vi "_Get App Ref from Info.vi"(8 "error in (no error)":errorcluster, 9 "Analysis App Info":T1) -> (0 "error out":errorcluster, 1 "Analysis App ref":refnum<vi>)   [LabVIEW 2017, in "CSM_ExampleBrowser.lvlib"]
uses:
  <vilib>/addons/analyzer/_analyzerctrls.llb/VIAnCtl Analysis App Info.ctl
  globals/User Visible Strings.vi
  CSM_ExampleBrowser.lvlib
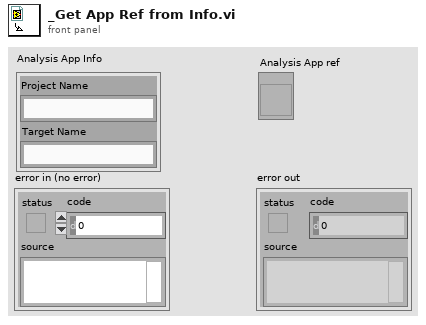
[diagram p1: front panel]
types:
  T1 = typedef "VIAnCtl Analysis App Info.ctl" = cluster{"Project Name":string, "Target Name":string}
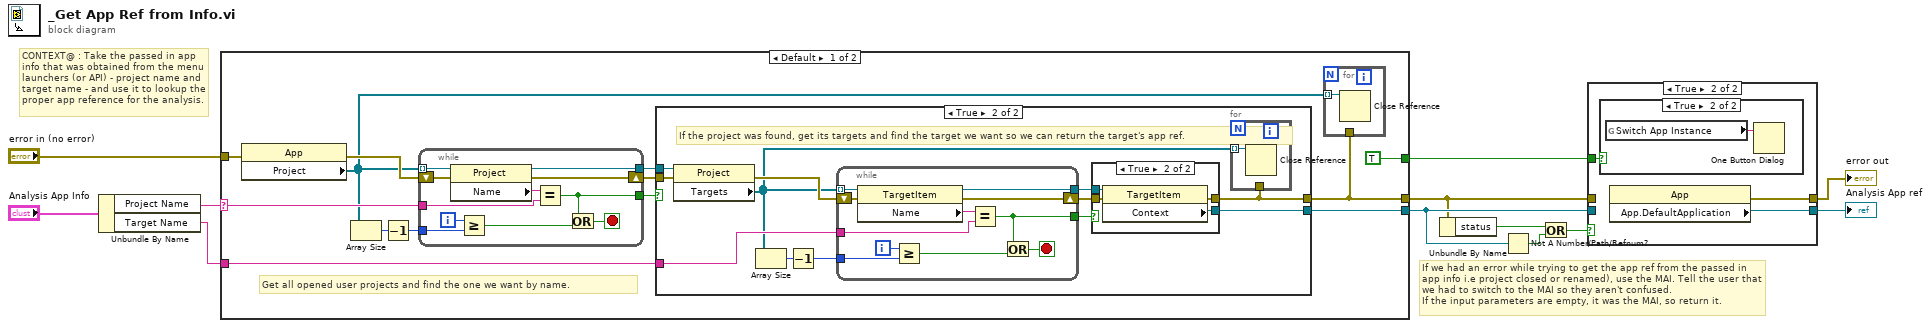
[diagram p0: block diagram]
diagram:
  # "If we had an error while trying to get the app ref from the passed in app info i.e project closed or renamed), use the MAI. Tell the user that we had to switch to the MAI so they aren't confused. \nIf the input parameters are empty, it was the MAI, so return it."
  # "CONTEXT@ : Take the passed in app info that was obtained from the menu launchers (or API) - project name and target name - and use it to lookup the proper app reference for the analysis."
  n1 = Unbundle By Name("Analysis App Info") -> ("Project Name"=w11:string, "Target Name"=w10:string)
  n2 = case shown="Default" w11 {
    selector: w11 -> [w22 _]
    tunnel: [w18 _] -> w6
    tunnel: w10 -> [w19 _]
    tunnel: [w14 _] -> w4
    tunnel: "error in (no error)" -> [w16 _]
    tunnel: [TRUE _] -> w1
    frame Default {
      # "Get all opened user projects and find the one we want by name."
      n3 = property class="App"(error in=w16) -> (error out=w23:errorcluster, "Project"=w17:refnum<vi>[])  [unwired: 1 in, 1 out]
      n4 = Array Size(array=w17) -> (size(s)=w25:i32)
      n5 = Decrement(x=w25) -> (x-1=w24:i32)
      n6 = while {
        tunnel: w17 -> [w65] mode=indexing
        tunnel: w24 -> [w67]
        shift-right: [w60] -> w20
        shift-left: w23 -> [w64]
        tunnel: w22 -> [w62]
        tunnel: [w61] -> w21
        tunnel: [w57] -> w15
        i -> [w66]
        stop <- w58 stop-if-true
        n7 = property class="Project"(reference=w65, error in=w64) -> (reference out=w61:refnum<vi>, error out=w60:errorcluster, "Name"=w63:string)
        n8 = Greater Or Equal?(x=w66, y=w67) -> (x >= y?=w59:bool)
        n9 = Equal?(x=w63, y=w62) -> (x = y?=w57:bool)
        n10 = Or(x=w57, y=w59) -> (x .or. y?=w58:bool)
      }
      n11 = case shown="True" w15 {
        tunnel: w21 -> [_ w38]
        tunnel: w20 -> [w26 w37]
        tunnel: w19 -> [_ w33]
        tunnel: [_ w30] -> w18
        tunnel: [w26 w28] -> w14
        frame False {
        }
        frame True {
          # "If the project was found, get its targets and find the target we want so we can return the target's app ref."
          n12 = property class="Project"(reference=w38, error in=w37) -> (error out=w34:errorcluster, "Targets"=w29:refnum<vi>[])  [unwired: 1 out]
          n13 = Array Size(array=w29) -> (size(s)=w36:i32)
          n14 = Decrement(x=w36) -> (x-1=w35:i32)
          n15 = while {
            tunnel: w29 -> [w53] mode=indexing
            tunnel: w35 -> [w55]
            shift-right: [w48] -> w31
            shift-left: w34 -> [w52]
            tunnel: w33 -> [w50]
            tunnel: [w49] -> w32
            tunnel: [w45] -> w27
            i -> [w54]
            stop <- w46 stop-if-true
            n16 = property class="TargetItem"(reference=w53, error in=w52) -> (reference out=w49:refnum<vi>, error out=w48:errorcluster, "Name"=w51:string)
            n17 = Greater Or Equal?(x=w54, y=w55) -> (x >= y?=w47:bool)
            n18 = Equal?(x=w51, y=w50) -> (x = y?=w45:bool)
            n19 = Or(x=w45, y=w47) -> (x .or. y?=w46:bool)
          }
          n20 = case shown="True" w27 {
            tunnel: w32 -> [_ w43]
            tunnel: w31 -> [w39 w42]
            tunnel: [_ w41] -> w30
            tunnel: [w39 w40] -> w28
            frame False {
            }
            frame True {
              n21 = property class="TargetItem"(reference=w43, error in=w42) -> (error out=w40:errorcluster, "Context"=w41:refnum<vi>)  [unwired: 1 out]
            }
          }
          n22 = for {
            tunnel: w29 -> [w44] mode=indexing
            tunnel: w28 -> [_]
            n23 = Close Reference(reference=w44) -> ()  [unwired: 1 in, 1 out]
          }
        }
      }
      n24 = for {
        tunnel: w17 -> [w56] mode=indexing
        tunnel: w14 -> [_]
        n25 = Close Reference(reference=w56) -> ()  [unwired: 1 in, 1 out]
      }
    }
    frame "" {
    }
  }
  n26 = Unbundle By Name(w4) -> ("status"=w8:bool)
  n27 = Not A Number/Path/Refnum?(number/path/refnum=w6) -> (NaN/Path/Refnum?=w7:bool)
  n28 = Or(x=w8, y=w7) -> (x .or. y?=w5:bool)
  n29 = case shown="True" w5 {
    tunnel: w6 -> [w68 _]
    tunnel: w4 -> [_ _]
    tunnel: [w68 w71] -> w3
    tunnel: [_ w70] -> w2
    tunnel: w1 -> [_ w69]
    frame False {
    }
    frame True {
      n30 = case shown="True" w69 {
        frame False {
        }
        frame True {
          n31 = global read "User Visible Strings.vi" "Switch App Instance"() -> (w72:string)
          n32 = One Button Dialog(message=w72) -> ()  [unwired: 2 out]
        }
      }
      n33 = property class="App"() -> (error out=w70:errorcluster, "App.DefaultApplication"=w71:refnum<vi>)  [unwired: 2 in, 1 out]
    }
  }
  "Analysis App ref" <- w3
  "error out" <- w2
